vi "Wrong_Address.vi"(1 "Software Address":i32, 2 "Hardware Address":i32) -> (0 "New Software Address":i32)   [LabVIEW 2011]
doc: "This VI is called from \"Start USB\". This is a prompt for the user if the USB address of the connected hardware does not match the address stored in file \"USB_DAQ.ini\"."
panel:
  in  "Change Software Address":bool
  in  "Abort":bool
  in  "Hardware Address 2":i32
  out "Software Address2":i32 format="%x"
  out "Hardware Address2":i32 format="%x"
  # "Wrong Address!"
  # "Hardware Address:"
  # "The software address:"
  # "Do you want to change the software address setting to match hardware or \"abort\"?"
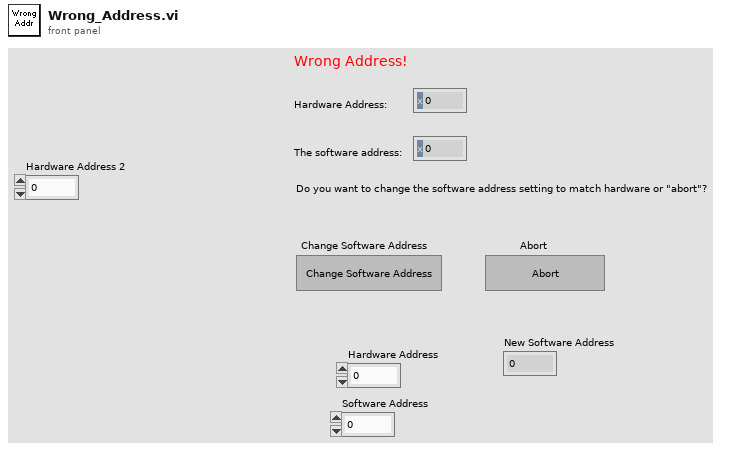
[diagram p1: front panel]
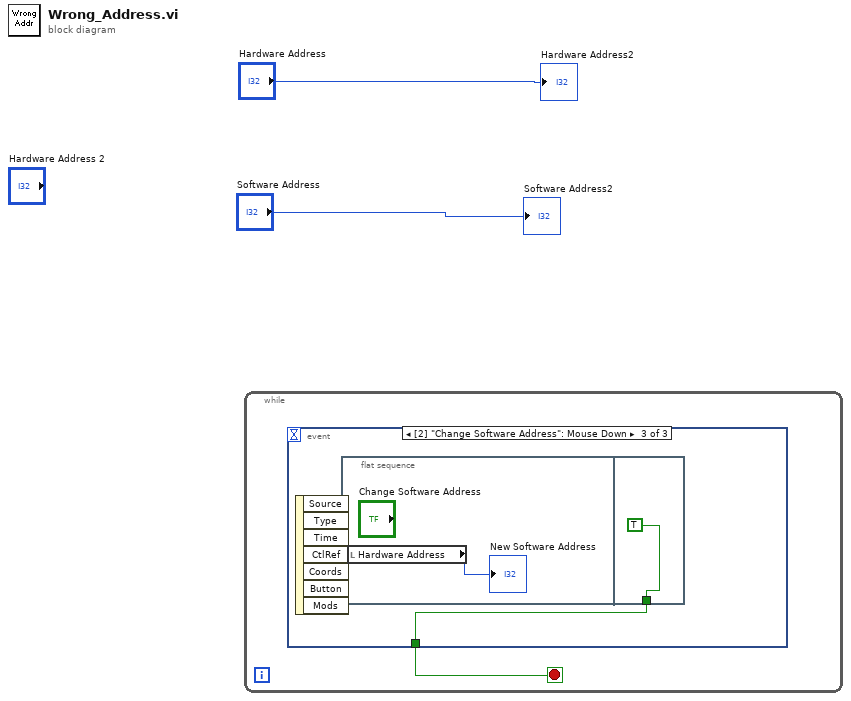
[diagram p0: block diagram]
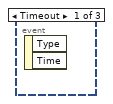
[diagram p2: hidden frame]
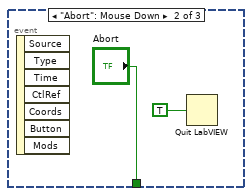
[diagram p3: hidden frame]
diagram:
  n1 = while {
    stop <- w3 stop-if-true
    n2 = event shown="[2] \"Change Software Address\": Mouse Down" {
      selector: _ -> [_ _ _]
      dyn-events: _ -> [_ _ _]
      timeout: _ -> [_ _ _]
      tunnel: [_ "Abort" w6] -> w3
      event Timeout {
        n3 = event-data() -> ()  [unwired: 1 in, 2 out]
      }
      event "Abort": Mouse Down {
        n4 = event-data() -> ()  [unwired: 1 in, 7 out]
        n5 = Quit LabVIEW(quit? (T)=TRUE) -> ()
      }
      event "Change Software Address": Mouse Down {
        n6 = event-data() -> ()  [unwired: 1 in, 7 out]
        n7 = flat-sequence {
          tunnel: [TRUE] -> w6
          frame #0 {
            n8 = local read "Hardware Address"() -> (→"New Software Address":i32)
          }
          frame #1 {
          }
        }
      }
    }
  }
  "Hardware Address2" <- "Hardware Address"
  "Software Address2" <- "Software Address"
